vi "Configure Sequence.vi"(8 "error in (no error)":errorcluster, 9 "Active Steps (0000000000)":bool[](array[boolean]), 10 "Sequence Number (1)":dbl=1.0 min=1.0 max=10.0 step=1.0 format="%#.0p", 11 "VISA resource name":refnum<visa-resource-name>) -> (0 "error out":errorcluster, 3 "VISA resource name out":refnum<visa-resource-name>)   [LabVIEW 2020, in "BK Precision 911X Series.lvlib"]
doc: "Selects the sequence to edit and configures a sequence's active steps. This VI should be used to select the steps to be active first, prior to running <b>Configure Sequence Parameters.vi</b> to configure the step parameters within the sequence.\n\n<b>Note: Sequence function is not supported for model 9117.</b>"
uses:
  BK Precision 911X Series.lvlib
panel:
  # "Steps   #  1   2    3   4    5   6   7    8   9   0"
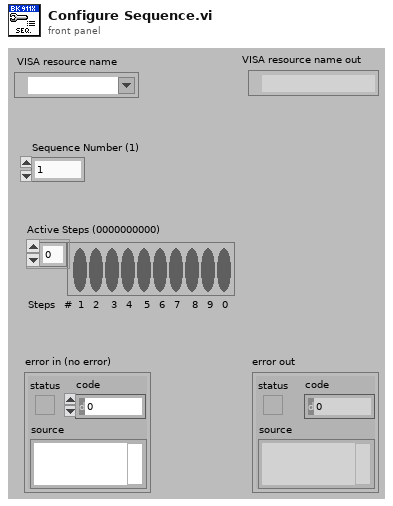
[diagram p1: front panel]
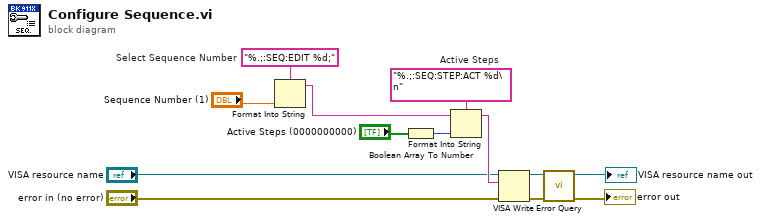
[diagram p0: block diagram]
diagram:
  w1 = "%.;:SEQ:STEP:ACT %d\n"  # Active Steps
  w2 = "%.;:SEQ:EDIT %d;"  # Select Sequence Number
  n1 = Format Into String(format string=w2, "Sequence Number (1)") -> (resulting string=w5:string)  [unwired: 2 in, 1 out]
  n2 = Boolean Array To Number(Boolean array="Active Steps (0000000000)") -> (number=w7:u32)
  n3 = Format Into String(format string=w1, initial string=w5, w7) -> (resulting string=w8:string)  [unwired: 1 in, 1 out]
  n4 = VISA Write(VISA resource name="VISA resource name", write buffer=w8, error in (no error)="error in (no error)") -> (VISA resource name out=w13:refnum<visa-resource-name>, error out=w12:errorcluster)  [unwired: 1 out]
  n5 = call "Error Query.vi"("error in (no error)"=w12, "VISA resource name"=w13) -> ("error out"=→"error out":errorcluster, "VISA resource name out"=→"VISA resource name out":refnum<visa-resource-name>)  [unwired: 6 in, 2 out]
